vi "GetCommonRef.vi"(8 "error in (no error)":errorcluster, 11 "FpgaRef5782 In":refnum<class "FpgaRefx410.lvclass">) -> (0 "error out":errorcluster, 2 "Common ref":T1, 3 "FpgaRef5782 Out":refnum<class "FpgaRefx410.lvclass">)   [LabVIEW 2025, in "FpgaRefx410.lvclass"]
uses:
  FpgaRefx410.lvclass
  FpgaRefBase/Common FPGA ref.ctl
  FpgaRefx410.lvclass/FpgaRefx410.ctl
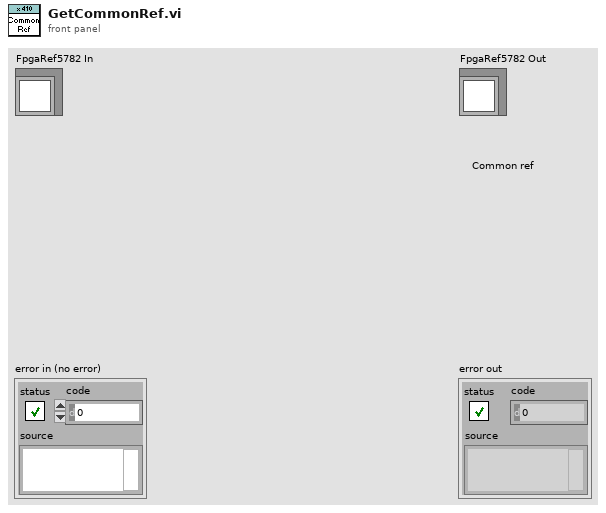
[diagram p1: front panel]
types:
  T1 = typedef "Common FPGA ref.ctl" = refnum<k20>
  T2 = typedef "x410 FPGA ref.ctl" = refnum<k20>
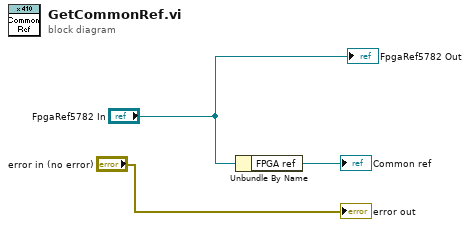
[diagram p0: block diagram]
diagram:
  n1 = Unbundle By Name("FpgaRef5782 In") -> ("FPGA ref"=→"Common ref":T2)
  "error out" <- "error in (no error)"
  "FpgaRef5782 Out" <- "FpgaRef5782 In"
